vi "tool_Unicode_Resize String Control.vi"(7 "Padding (10x5)":T1={"Width"=10, "Height"=5}, 8 "error in (no error)":errorcluster, 9 "Min Size (10x10)":T1={"Width"=10, "Height"=10}, 10 "Max Size (300x300)":T1={"Width"=300, "Height"=300}, 11 "*StrControl in":refnum<vi>) -> (0 "error out":errorcluster, 3 "*StrControl out":refnum<vi>)   [LabVIEW 2013, in "SET_Unicode Tools.lvlib"]
doc: "tool_Unicode_Resize String Control.vi\n\nPerform size to fit on a string control ref with given Max size, Min size,\nand padding. Units are pixels.\n\nScroll bar is set to visible if text is larger than Max Size."
uses:
  SET_Unicode Tools.lvlib
  <vilib>/Utility/miscctls.llb/LVBoundsTypeDef.ctl
panel:
  out "String Buffer":string
  out "Calculated Size":T1
  # "tool_Unicode_Resize String Control.vi\n\nPerform size to fit on a string control ref with given Max size, Min size,\nand padding. Units are pixels.\n\nScroll bar is set to visible if text is larger than Max Size."
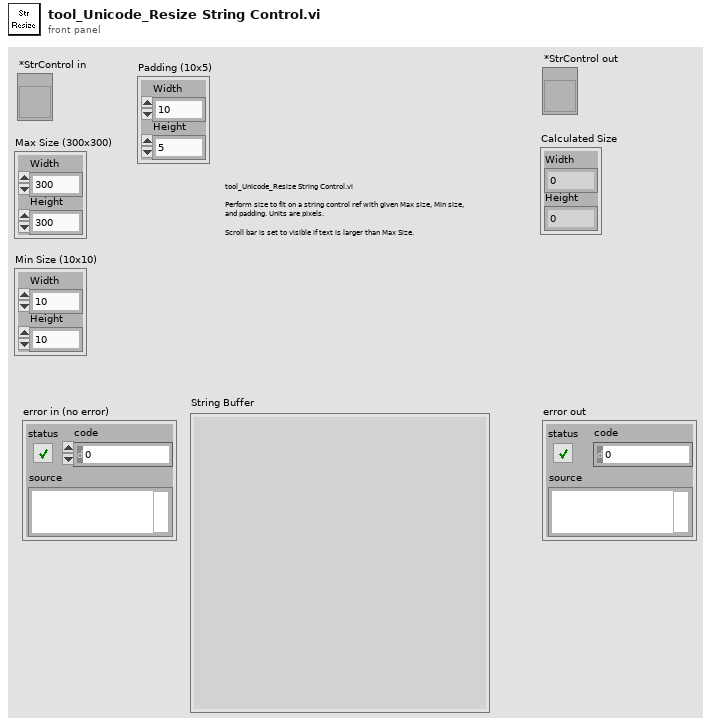
[diagram p1: front panel]
types:
  T1 = typedef "LVBoundsTypeDef.ctl" = cluster{"Width":u32, "Height":u32}
  T2 = typedef "LVFontTypeDef.ctl" = cluster{"Font Name":string, "Size":u16, "Bold":bool, "Italic":bool, "Underline":bool, "Strikeout":bool, "Color":u32}
  T3 = cluster{"Font Name:":string, "Size":i16, "Strikeout?":bool, "Italic?":bool, "Underline?":bool, "Outline?":bool, "Shadow?":bool, "Bold?":bool}
  T4 = enum16{"None", "Stacked", "Clockwise", "Counterclockwise"}
  T5 = enum16{"User-specified Font", "Application Font", "System Font", "Dialog Font"}
  T6 = cluster{"left":i16, "top":i16, "right":i16, "bottom":i16}
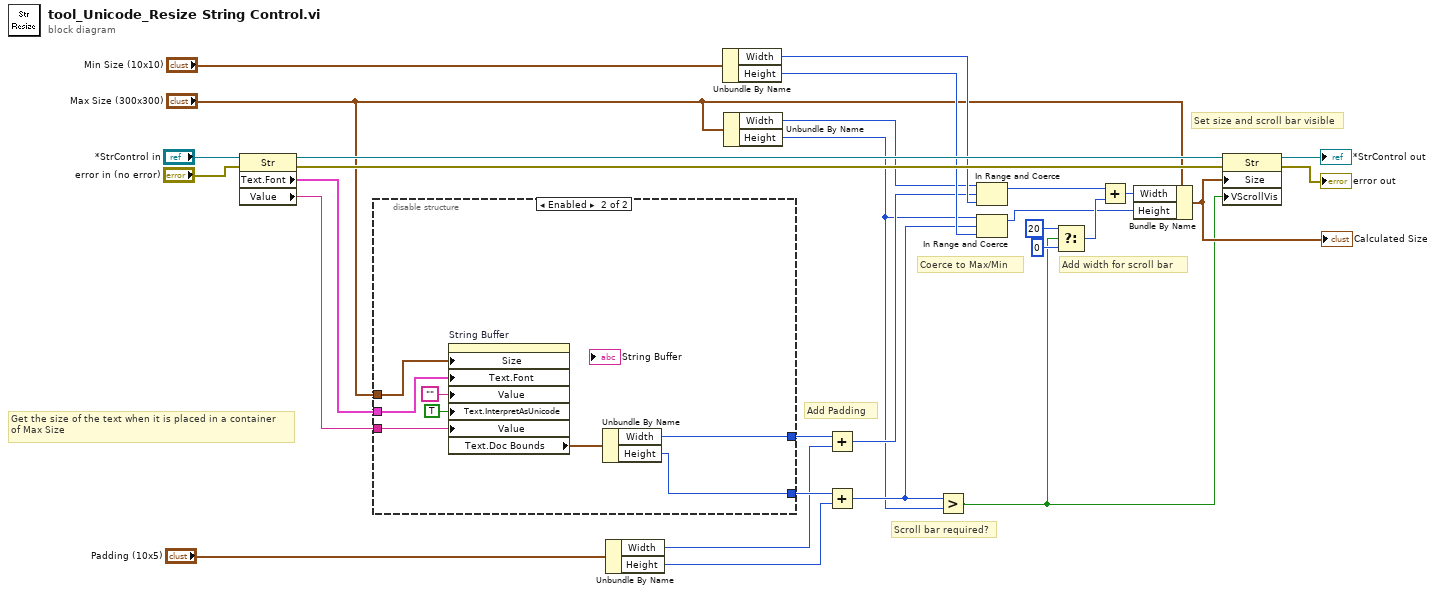
[diagram p0: block diagram]
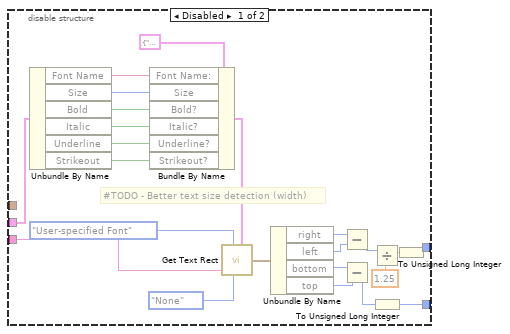
[diagram p2: hidden frame]
diagram:
  # "Get the size of the text when it is placed in a container\nof Max Size"
  # "Add Padding"
  # "Scroll bar required?"
  # "Add width for scroll bar"
  # "Coerce to Max/Min"
  # "Set size and scroll bar visible"
  n1 = property class="Str"(reference="*StrControl in", error in="error in (no error)") -> (reference out=w16:refnum<vi>, error out=w26:errorcluster, "Text.Font"=w29:T2, "Value"=w17:string)
  n2 = disable-structure shown="Enabled" {
    disable-tunnel: w29 -> [w51 w57]
    disable-tunnel: [w40 w60] -> w10
    disable-tunnel: [w39 w59] -> w23
    disable-tunnel: w17 -> [w38 w54]
    disable-tunnel: "Max Size (300x300)" -> [_ w58]
    frame Disabled {
      # "#TODO - Better text size detection (width)"
      n3 = Unbundle By Name(w51) -> ("Font Name"=w49:string, "Size"=w48:u16, "Bold"=w47:bool, "Italic"=w44:bool, "Underline"=w45:bool, "Strikeout"=w43:bool)
      n4 = Bundle By Name(cluster=T3 {"Font Name:"="", "Size"=0, "Strikeout?"=FALSE, "Italic?"=FALSE, "Underline?"=FALSE, "Outline?"=FALSE, "Shadow?"=FALSE, "Bold?"=FALSE} ("[user-specified font]"), "Font Name:"=w49, "Size"=w48, "Bold?"=w47, "Italic?"=w44, "Underline?"=w45, "Strikeout?"=w43) -> (w46:T3)
      n5 = call <vilib>:"Get Text Rect.vi"("desired font(Application)"=T5."User-specified Font", "text"=w38, "text orientation"=T4."None", "[user-specified font]"=w46) -> ("rect"=w52:T6)  [unwired: 5 in]
      n6 = Unbundle By Name(w52) -> ("right"=w37:i16, "left"=w36:i16, "bottom"=w34:i16, "top"=w35:i16)
      n7 = Subtract(x=w37, y=w36) -> (x-y=w33:i16)
      n8 = Subtract(x=w34, y=w35) -> (x-y=w30:i16)
      n9 = Divide(x=w33, y=1.25) -> (x/y=w31:dbl)
      n10 = To Unsigned Long Integer(number=w30) -> (unsigned 32bit integer=w39:u32)
      n11 = To Unsigned Long Integer(number=w31) -> (unsigned 32bit integer=w40:u32)
    }
    frame Enabled {
      n12 = property on="String Buffer" class="Str"("Size"=w58, "Text.Font"=w57, "Value"="", "Text.InterpretAsUnicode"=TRUE ("Text.Interpret As Unicode"), "Value"=w54) -> ("Text.Doc Bounds"=w53:T1)  [unwired: 2 in, 2 out]
      n13 = Unbundle By Name(w53) -> ("Width"=w60:u32, "Height"=w59:u32)
    }
  }
  n14 = Unbundle By Name("Padding (10x5)") -> ("Width"=w7:u32, "Height"=w6:u32)
  n15 = Unbundle By Name("Min Size (10x10)") -> ("Width"=w14:u32, "Height"=w12:u32)
  n16 = Unbundle By Name("Max Size (300x300)") -> ("Width"=w11:u32, "Height"=w2:u32)
  n17 = Add(x=w10, y=w7) -> (x+y=w4:u32)
  n18 = Add(x=w23, y=w6) -> (x+y=w3:u32)
  n19 = Greater?(x=w3, y=w2) -> (0:w1:bool)
  n20 = In Range and Coerce(upper limit=w11, x=w4, lower limit=w14) -> (coerced(x)=w13:u32)  [unwired: 1 out]
  n21 = In Range and Coerce(upper limit=w2, x=w3, lower limit=w12) -> (coerced(x)=w5:u32)  [unwired: 1 out]
  n22 = Select(t=u32 20 ("y"), s=w1, f=u32 0 ("y")) -> (s? t:f=w19:u32)
  n23 = Add(x=w13, y=w19) -> (x+y=w18:u32)
  n24 = Bundle By Name(cluster="Max Size (300x300)", "Width"=w18, "Height"=w5) -> (w22:T1)
  "Calculated Size" <- w22
  n25 = property class="Str"(reference=w16, error in=w26, "Size"=w22, "VScrollVis"=w1) -> (reference out=→"*StrControl out":refnum<vi>, error out=→"error out":errorcluster)
